vi "avg of n random nos using stack.vi"() -> ()   [LabVIEW 2018]
panel:
  in  "Numeric 2":i32
  out "Numeric":dbl
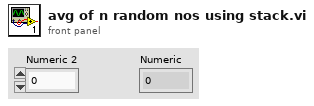
[diagram p1: front panel]
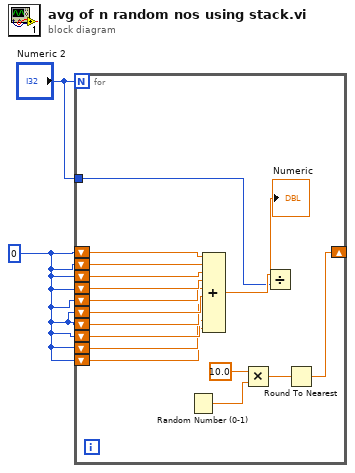
[diagram p0: block diagram]
diagram:
  w2 = 0
  n1 = for {
    N: "Numeric 2" -> [_]
    shift-right: [w6] -> _
    shift-left: w2 -> [w19]
    shift-left: w2 -> [w18]
    shift-left: w2 -> [w17]
    shift-left: w2 -> [w16]
    shift-left: w2 -> [w15]
    shift-left: w2 -> [w14]
    shift-left: w2 -> [w13]
    shift-left: w2 -> [w12]
    shift-left: w2 -> [w11]
    shift-left: w2 -> [w10]
    tunnel: "Numeric 2" -> [w4]
    n2 = Random Number (0-1)() -> (number: 0 to 1=w9:dbl)
    n3 = Compound Arithmetic op=ADD(w19, w18, w17, w16, w15, w14, w13, w12, w11, w10) -> (w5:dbl)
    n4 = Multiply(x=10.0, y=w9) -> (x*y=w7:dbl)
    n5 = Divide(x=w5, y=w4) -> (x/y=→"Numeric":dbl)
    n6 = Round To Nearest(number=w7) -> (nearest integer value=w6:dbl)
  }
